vi "Arm Tasks.vi"(1 "Arm Movement Parameters":T1) -> ()   [LabVIEW 2015]
uses:
  Robot Global Data.vi
  <vilib>/Rock Robotics/Network Tables/NT Write Number.vi
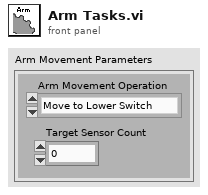
[diagram p1: front panel]
types:
  T1 = cluster{"Arm Movement Operation":enum16{"Move to Lower Switch", "Move to Upper Switch", "Move to Sensor Count"}, "Target Sensor Count":i32}
  T2 = enum16{"Move to Lower Switch", "Move to Upper Switch", "Move to Sensor Count"}
  T3 = typedef "WPI_SwitchDevRef.ctl" = cluster{"DevStatus":errorcluster, "DIO Channel":T4, "CntIndex":T5, "Normally Closed":bool}
  T4 = typedef "FPGA_DIOChannel.ctl" = enum8{"DIO 0", "DIO 1", "DIO 2", "DIO 3", "DIO 4", "DIO 5", "DIO 6", "DIO 7", "DIO 8", "DIO 9", "DIO MXP 0", "DIO MXP 1", "DIO MXP 2", "DIO MXP 3", "DIO MXP 4", "DIO MXP 5", "DIO MXP 6", "DIO MXP 7", "DIO MXP 8", "DIO MXP 9", "DIO MXP 10", "DIO MXP 11", "DIO MXP 12", "DIO MXP 13", "DIO MXP 14", "DIO MXP 15", "Invalid"}
  T5 = typedef "FPGA_CounterCtrSystemIndex.ctl" = enum8{"Ctr 0", "Ctr 1", "Ctr 2", "Ctr 3", "Ctr 4", "Ctr 5", "Ctr 6", "Ctr 7", "Invalid"}
  T6 = typedef "WPI_MotorControlDeviceRef.ctl" = cluster{"DeviceStatus":errorcluster, "Type":T7, "PWM":cluster{"PWM Channel":T8, "DeadBand":T9}, "CAN":cluster{"Device Number":u8, "Control Mode":T10, "Semaphore":T11, "Max Vout":dbl, "TalonSRX Control Mode":T12}, "Invert":bool}
  T7 = typedef "WPI_MotorControlType.ctl" = enum16{"PWM", "CAN", "CANTalonSRX"}
  T8 = typedef "FPGA_DIOPWMChannel.ctl" = enum8{"PWM 0", "PWM 1", "PWM 2", "PWM 3", "PWM 4", "PWM 5", "PWM 6", "PWM 7", "PWM 8", "PWM 9", "PWM MXP 0", "PWM MXP 1", "PWM MXP 2", "PWM MXP 3", "PWM MXP 4", "PWM MXP 5", "PWM MXP 6", "PWM MXP 7", "PWM MXP 8", "PWM MXP 9", "Invalid"}
  T9 = typedef "WPI_PWMDeadband.ctl" = cluster{"Name":string, "maxPositivePwm":i32, "minPositivePwm":i32, "centerPwm":i32, "maxNegativePwm":i32, "minNegativePwm":i32, "angularRange":u16}
  T10 = typedef "WPI_CANJaguar_ControlMode.ctl" = enum8{"Percent VBus", "Current", "Speed", "Position", "Voltage"}
  T11 = typedef "Semaphore RefNum" = refnum<k1>
  T12 = typedef "WPI_CANTalonSRX_APIControlMode.ctl" = enum8{"Percent VBus", "Speed", "Position", "Slave", "Unchanged / Invalid", "Voltage Compensation", "Current", "Motion Profile"}
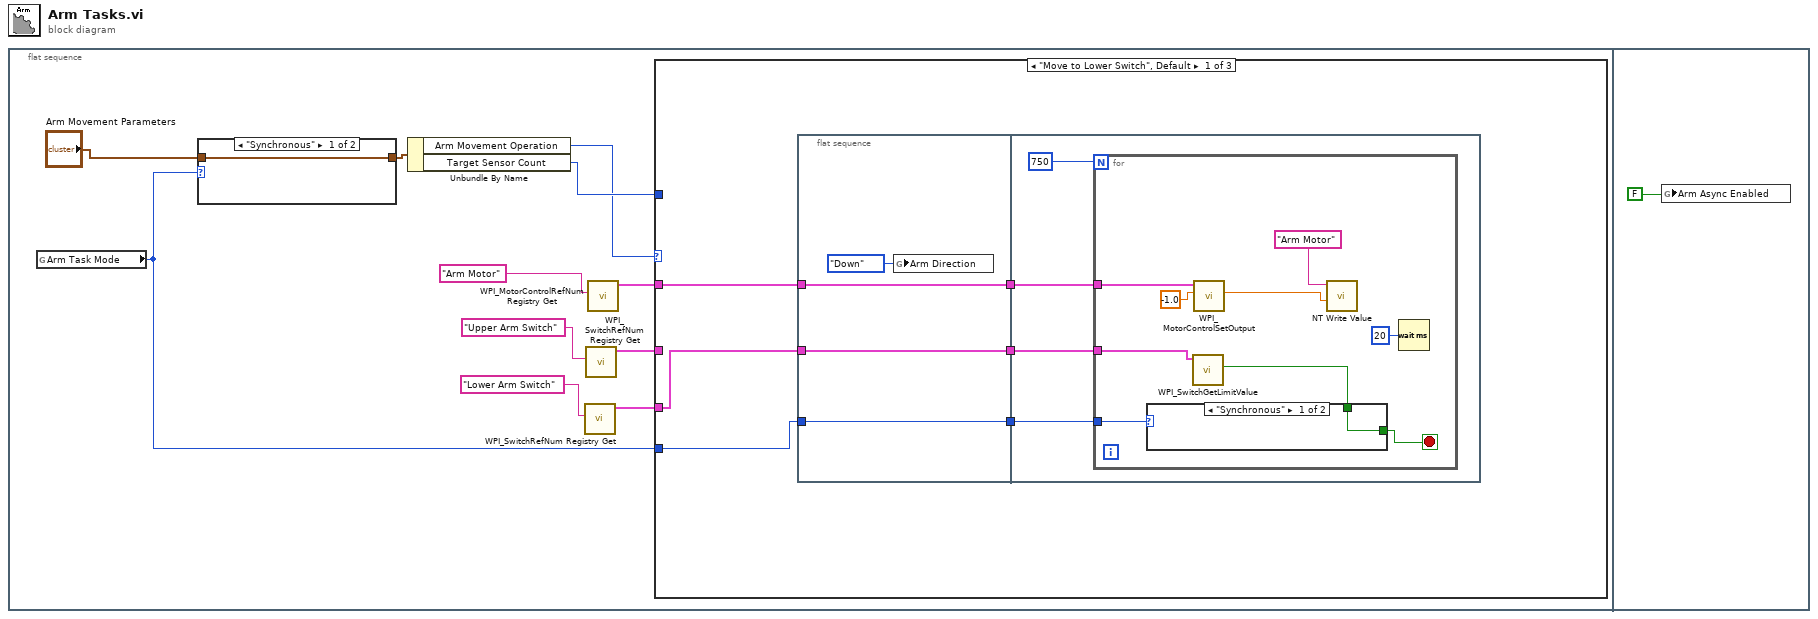
[diagram p0: block diagram]
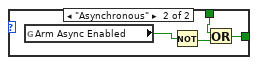
[diagram p2: hidden frame]
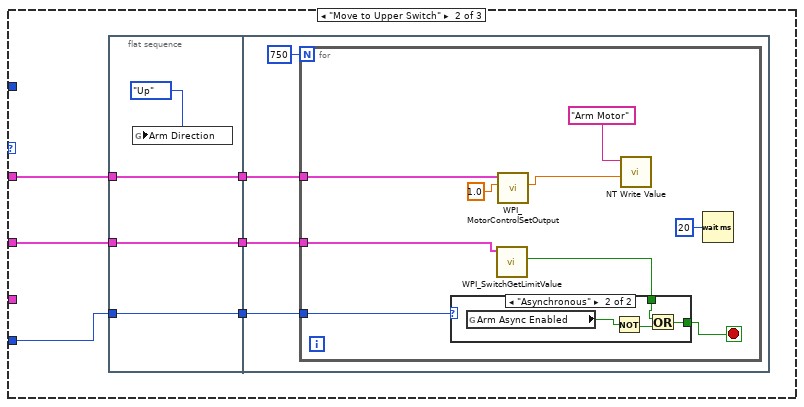
[diagram p3: hidden frame]
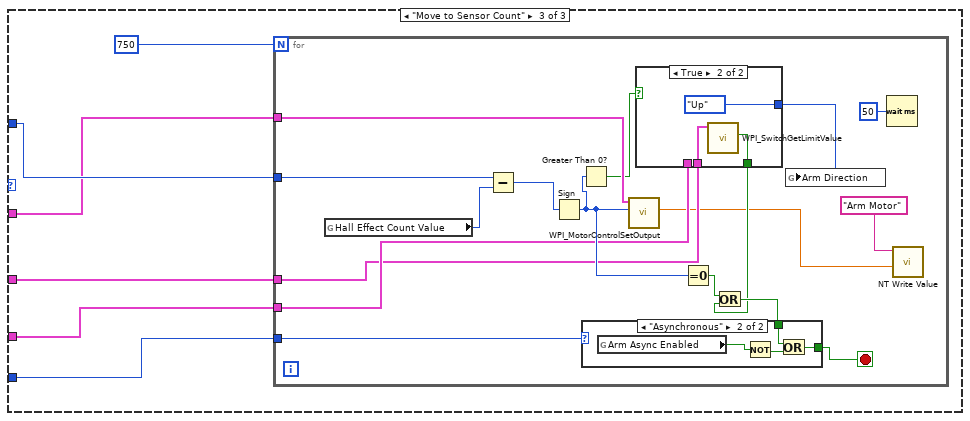
[diagram p5: hidden frame]
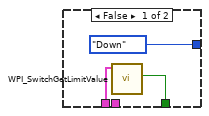
[diagram p6: hidden frame]
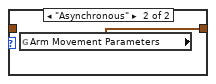
[diagram p8: hidden frame]
diagram:
  n1 = flat-sequence {
    frame #0 {
      n2 = global read "Robot Global Data.vi" "Arm Task Mode"() -> (w10:enum16{"Synchronous", "Asynchronous"})
      n3 = case shown="\"Synchronous\"" w10 {
        tunnel: [w102 w103] -> w8
        tunnel: "Arm Movement Parameters" -> [w102 _]
        frame "Synchronous" {
        }
        frame "Asynchronous" {
          n4 = global read "Robot Global Data.vi" "Arm Movement Parameters"() -> (w103:T1)
        }
      }
      n5 = Unbundle By Name(w8) -> ("Arm Movement Operation"=w9:T2, "Target Sensor Count"=w11:i32)
      n6 = call <vilib>:"WPI_SwitchRefNum Registry Get.vi"("refnum name"="Lower Arm Switch") -> ("SwitchDevRef"=w4:T3)  [unwired: 9 in, 1 out]
      n7 = call <vilib>:"WPI_SwitchRefNum Registry Get.vi"("refnum name"="Upper Arm Switch") -> ("SwitchDevRef"=w6:T3)  [unwired: 9 in, 1 out]
      n8 = call <vilib>:"WPI_MotorControlRefNum Registry Get.vi"("refnum name"="Arm Motor") -> ("MotorControlDevRef"=w2:T6)  [unwired: 9 in, 1 out]
      n9 = case shown="\"Move to Lower Switch\", Default" w9 {
        tunnel: w11 -> [_ _ w72]
        tunnel: w10 -> [w15 w45 w73]
        tunnel: w6 -> [_ w44 w71]
        tunnel: w4 -> [w16 _ w70]
        tunnel: w2 -> [w17 w43 w68]
        frame "Move to Lower Switch", Default {
          n10 = flat-sequence {
            tunnel: w15 -> [w19]
            tunnel: w16 -> [w20]
            tunnel: w17 -> [w21]
            tunnel: [w21] -> w14
            tunnel: [w20] -> w13
            tunnel: [w19] -> w12
            tunnel: w14 -> [w25]
            tunnel: w13 -> [w24]
            tunnel: w12 -> [w23]
            frame #0 {
              n11 = global write "Robot Global Data.vi" "Arm Direction"(enum16{"Up", "Down"}."Down" ("Arm Direction")) -> ()
            }
            frame #1 {
              n12 = for {
                N: 750 -> [_]
                tunnel: w23 -> [w34]
                tunnel: w24 -> [w32]
                tunnel: w25 -> [w29]
                stop <- w33 stop-if-true
                n13 = call <vilib>:"WPI_SwitchGetLimitValue.vi"("SwitchDevRef"=w32) -> ("Switch Pressed"=w31:bool)  [unwired: 8 in, 2 out]
                n14 = case shown="\"Synchronous\"" w34 {
                  tunnel: [w35 w38] -> w33
                  tunnel: w31 -> [w35 w37]
                  frame "Synchronous" {
                  }
                  frame "Asynchronous" {
                    n15 = global read "Robot Global Data.vi" "Arm Async Enabled"() -> (w39:bool)
                    n16 = Not(x=w39) -> (.not. x?=w36:bool)
                    n17 = Or(x=w37, y=w36) -> (x .or. y?=w38:bool)
                  }
                }
                n18 = call <vilib>:"WPI_MotorControlSetOutput.vi"("Output"=-1.0, "MotorControlDevRef"=w29) -> ("Motor Output"=w26:dbl)  [unwired: 7 in, 2 out]
                n19 = call-poly <vilib>:"NT Write Value.vi"("Numeric"=w26, "Name"="Arm Motor") -> ()  [unwired: 9 in, 1 out]
                n20 = Wait (ms)(milliseconds to wait=u32 20) -> ()  [unwired: 1 out]
              }
            }
          }
        }
        frame "Move to Upper Switch" {
          n21 = flat-sequence {
            tunnel: w43 -> [w47]
            tunnel: w44 -> [w48]
            tunnel: w45 -> [w49]
            tunnel: [w49] -> w42
            tunnel: [w48] -> w41
            tunnel: [w47] -> w40
            tunnel: w42 -> [w53]
            tunnel: w41 -> [w52]
            tunnel: w40 -> [w50]
            frame #0 {
              n22 = global write "Robot Global Data.vi" "Arm Direction"(enum16{"Up", "Down"}."Up" ("Arm Direction")) -> ()
            }
            frame #1 {
              n23 = for {
                N: 750 -> [_]
                tunnel: w53 -> [w62]
                tunnel: w52 -> [w60]
                tunnel: w50 -> [w57]
                stop <- w61 stop-if-true
                n24 = call <vilib>:"WPI_SwitchGetLimitValue.vi"("SwitchDevRef"=w60) -> ("Switch Pressed"=w59:bool)  [unwired: 8 in, 2 out]
                n25 = case shown="\"Asynchronous\"" w62 {
                  tunnel: [w63 w66] -> w61
                  tunnel: w59 -> [w63 w65]
                  frame "Synchronous" {
                  }
                  frame "Asynchronous" {
                    n26 = global read "Robot Global Data.vi" "Arm Async Enabled"() -> (w67:bool)
                    n27 = Not(x=w67) -> (.not. x?=w64:bool)
                    n28 = Or(x=w65, y=w64) -> (x .or. y?=w66:bool)
                  }
                }
                n29 = call <vilib>:"WPI_MotorControlSetOutput.vi"("Output"=1.0, "MotorControlDevRef"=w57) -> ("Motor Output"=w54:dbl)  [unwired: 7 in, 2 out]
                n30 = call-poly <vilib>:"NT Write Value.vi"("Numeric"=w54, "Name"="Arm Motor") -> ()  [unwired: 9 in, 1 out]
                n31 = Wait (ms)(milliseconds to wait=u32 20) -> ()  [unwired: 1 out]
              }
            }
          }
        }
        frame "Move to Sensor Count" {
          n32 = for {
            N: 750 -> [_]
            tunnel: w73 -> [w88]
            tunnel: w72 -> [w86]
            tunnel: w71 -> [w76]
            tunnel: w70 -> [w78]
            tunnel: w68 -> [w82]
            stop <- w90 stop-if-true
            n33 = global read "Robot Global Data.vi" "Hall Effect Count Value"() -> (w87:i32)
            n34 = Subtract(x=w86, y=w87) -> (x-y=w85:i32)
            n35 = Sign(1:w85) -> (0:w81:i32)
            n36 = Greater Than 0?(x=w81) -> (x > 0?=w79:bool)
            n37 = call <vilib>:"WPI_MotorControlSetOutput.vi"("Output"=w81, "MotorControlDevRef"=w82) -> ("Motor Output"=w74:dbl)  [unwired: 7 in, 2 out]
            n38 = case shown="True" w79 {
              tunnel: [enum16{"Up", "Down"}."Down" ("Arm Direction") enum16{"Up", "Down"}."Up" ("Arm Direction")] -> w80
              tunnel: w78 -> [w92 _]
              tunnel: [w91 w94] -> w77
              tunnel: w76 -> [_ w95]
              frame False {
                n39 = call <vilib>:"WPI_SwitchGetLimitValue.vi"("SwitchDevRef"=w92) -> ("Switch Pressed"=w91:bool)  [unwired: 8 in, 2 out]
              }
              frame True {
                n40 = call <vilib>:"WPI_SwitchGetLimitValue.vi"("SwitchDevRef"=w95) -> ("Switch Pressed"=w94:bool)  [unwired: 8 in, 2 out]
              }
            }
            n41 = Equal To 0?(x=w81) -> (x = 0?=w84:bool)
            n42 = Or(x=w84, y=w77) -> (x .or. y?=w83:bool)
            n43 = case shown="\"Asynchronous\"" w88 {
              tunnel: [w97 w100] -> w90
              tunnel: w83 -> [w97 w98]
              frame "Synchronous" {
              }
              frame "Asynchronous" {
                n44 = global read "Robot Global Data.vi" "Arm Async Enabled"() -> (w101:bool)
                n45 = Not(x=w101) -> (.not. x?=w99:bool)
                n46 = Or(x=w98, y=w99) -> (x .or. y?=w100:bool)
              }
            }
            n47 = global write "Robot Global Data.vi" "Arm Direction"(w80) -> ()
            n48 = Wait (ms)(milliseconds to wait=u32 50) -> ()  [unwired: 1 out]
            n49 = call-poly <vilib>:"NT Write Value.vi"("Numeric"=w74, "Name"="Arm Motor") -> ()  [unwired: 9 in, 1 out]
          }
        }
      }
    }
    frame #1 {
      n50 = global write "Robot Global Data.vi" "Arm Async Enabled"(FALSE) -> ()
    }
  }
